vi "MeasLeakRate13.vi"() -> ()   [LabVIEW 2011]
panel:
  out "error out":errorcluster
  out "fit":cluster{"element":dbl, "Value":dbl}[](array[cluster])
  out "T-T0,P":cluster{"element":dbl, "element":dbl}[](array[cluster])
  out "t0":dbl format="%#_8f"
  out "XY Graph":T1(graph)
  out "S00":i32
  out "S20":dbl
  out "S11":dbl
  out "S10":dbl
  out "S01":dbl
  out "T,P":cluster{"element":dbl, "element":dbl}[](array[cluster])
  out "dPdt":dbl
  out "P0":dbl
  out "average P (Torr)":string
  in  "Control Valve local":bool
  in  "Exhaust Local":bool
  in  "Exhaust Close":bool
  in  "Exhaust Open":bool
  in  "Control Close":bool
  in  "Control Open":bool
  in  "reset":bool
  in  "# points to watch":i32=60
  out "leak rate (Torr/min)":string
  out "P":dbl
  out "first":bool=TRUE
  in  "interval (s)":dbl=0.5
  in  "stop":bool
  out "P(Torr)":string
  # "Pressure control valve:"
  # "Exahaust valve:"
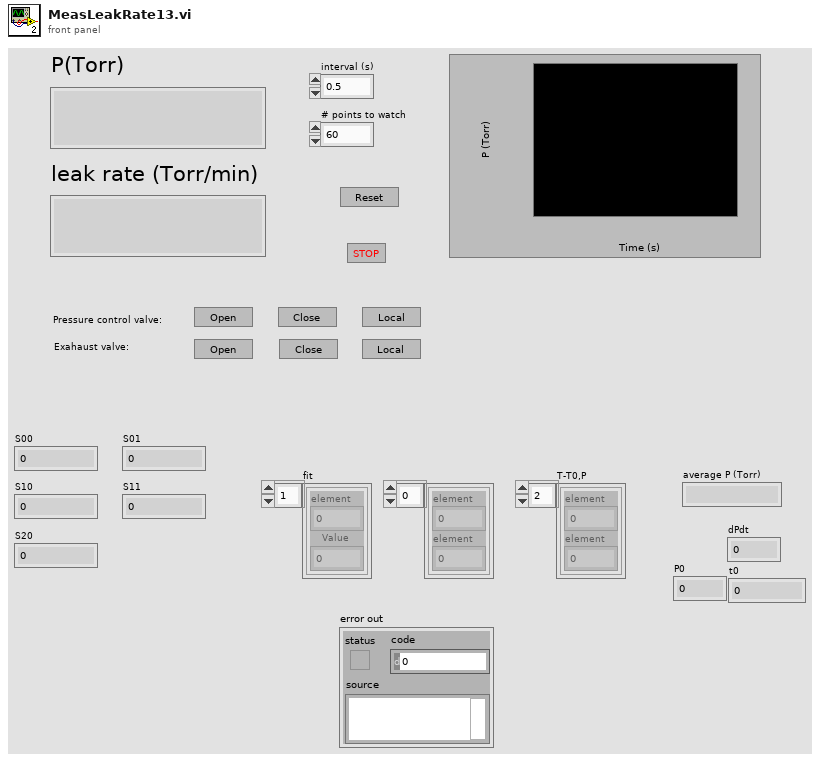
[diagram p1: front panel]
types:
  T1 = cluster{"Value":cluster{"element":dbl, "element":dbl}[]}[]
  T2 = cluster{"Value":cluster{"element":dbl, "Value":dbl}[]}[]
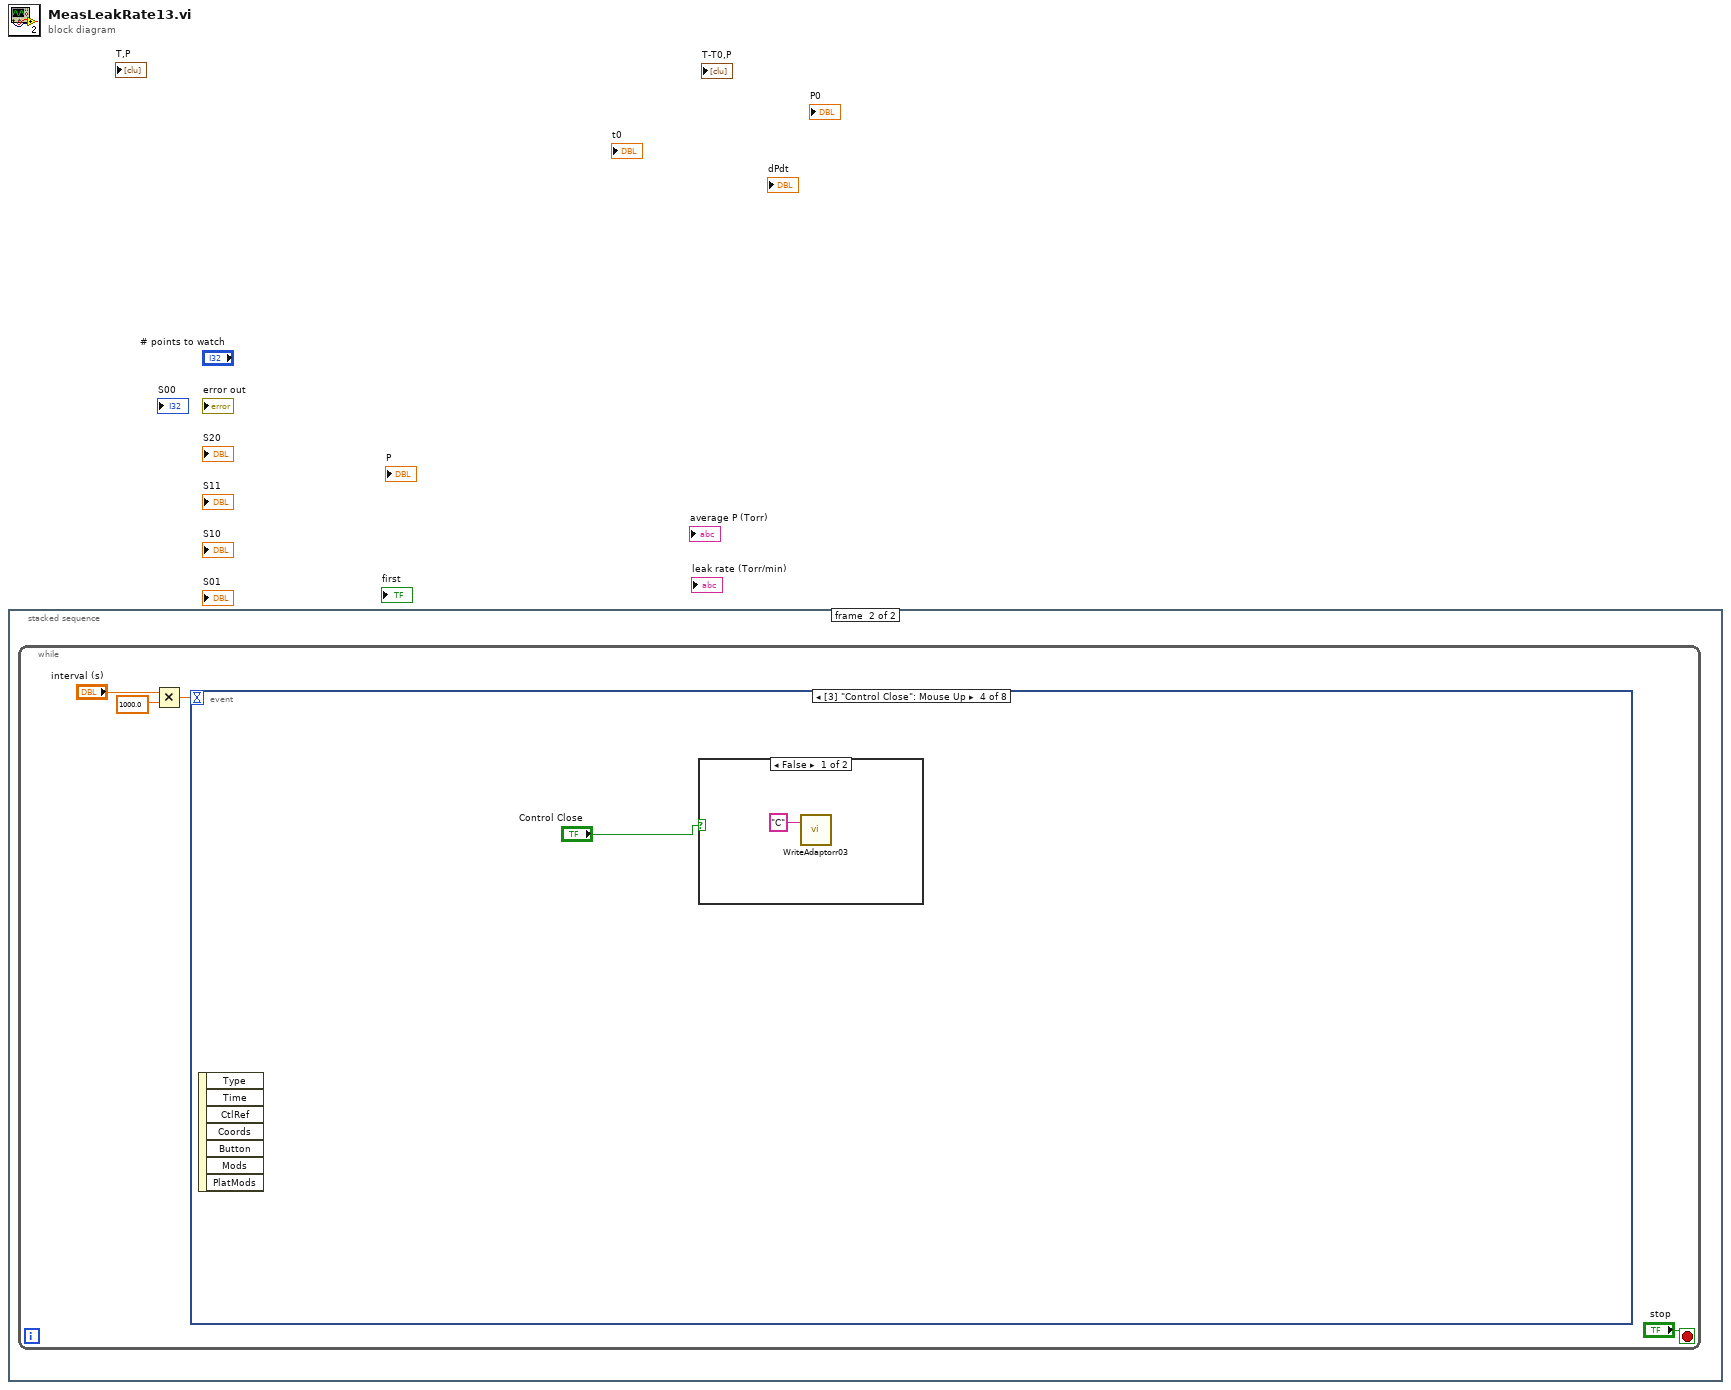
[diagram p0: block diagram]
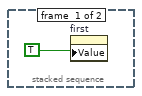
[diagram p2: hidden frame]
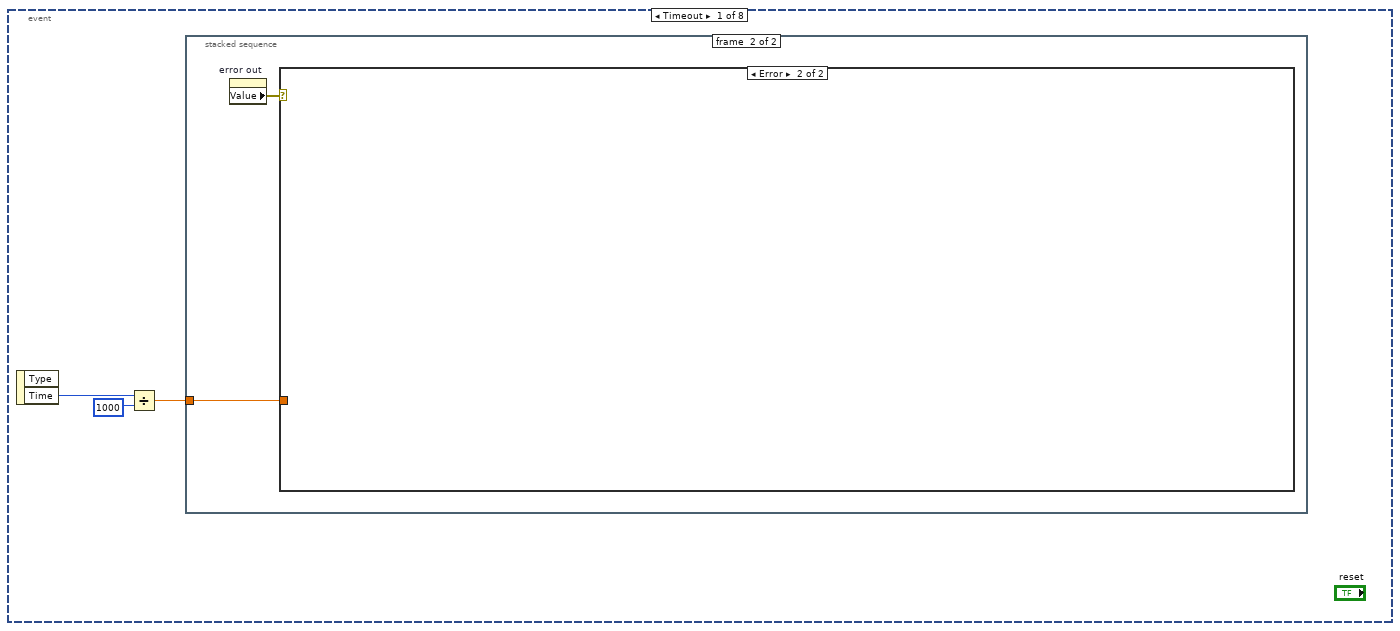
[diagram p3: hidden frame]
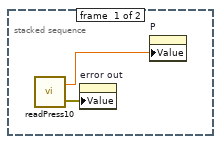
[diagram p4: hidden frame]
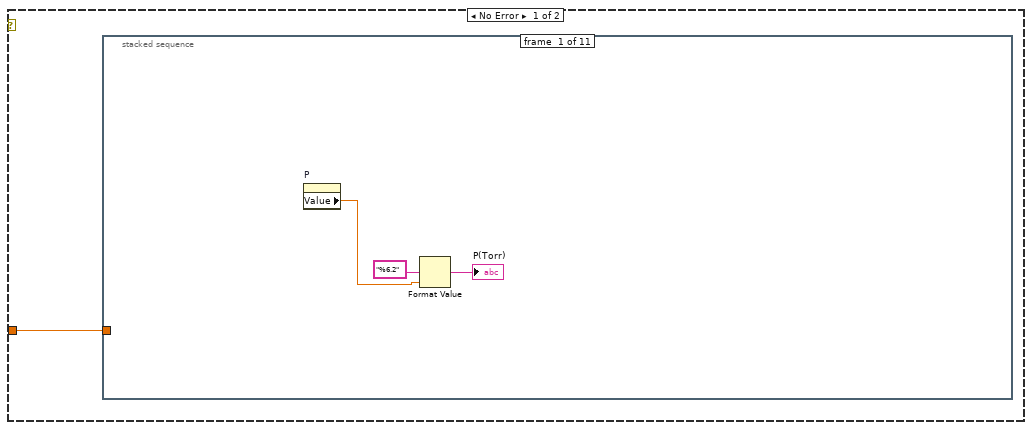
[diagram p5: hidden frame]
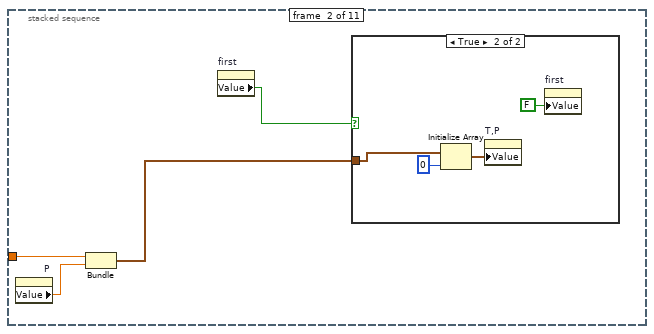
[diagram p6: hidden frame]
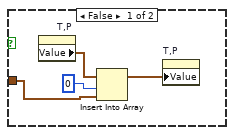
[diagram p7: hidden frame]
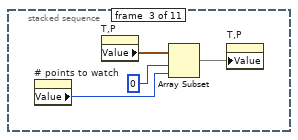
[diagram p8: hidden frame]
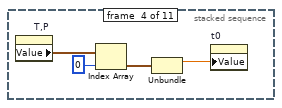
[diagram p9: hidden frame]
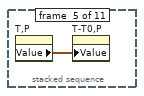
[diagram p10: hidden frame]
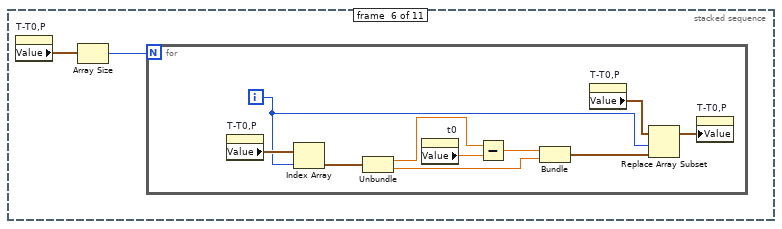
[diagram p11: hidden frame]
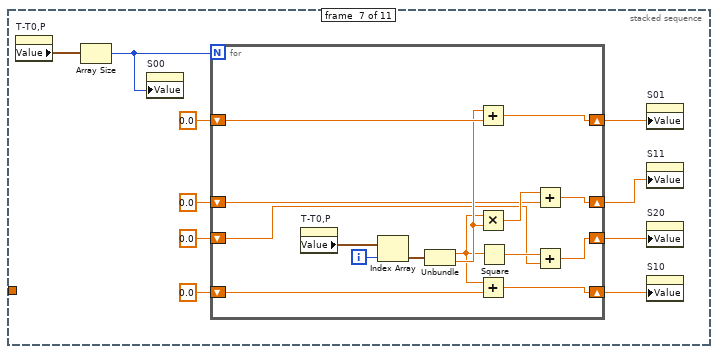
[diagram p12: hidden frame]
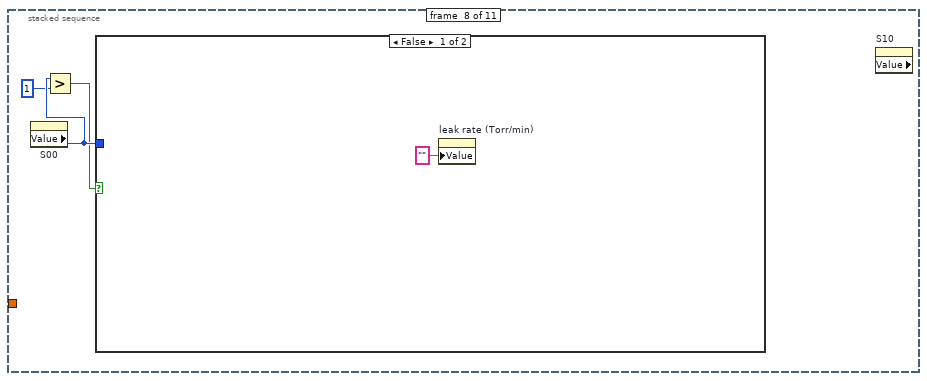
[diagram p13: hidden frame]
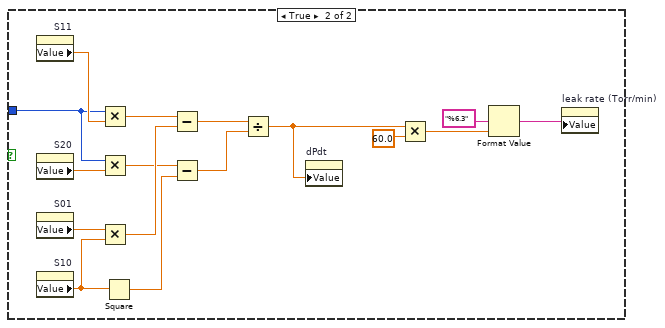
[diagram p14: hidden frame]
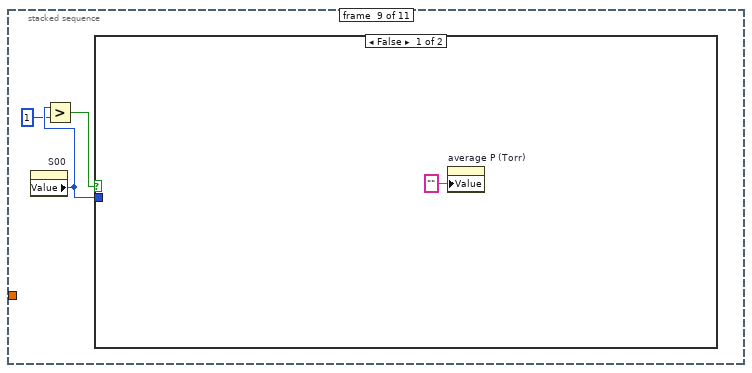
[diagram p15: hidden frame]
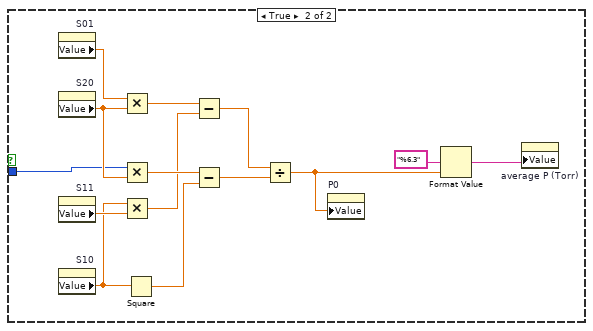
[diagram p16: hidden frame]
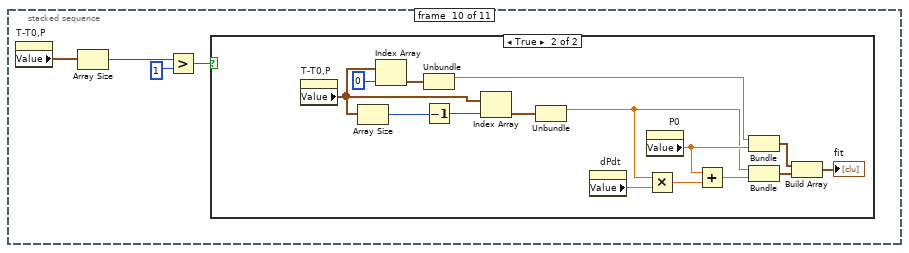
[diagram p17: hidden frame]
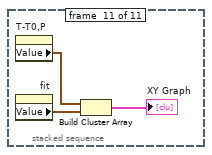
[diagram p19: hidden frame]
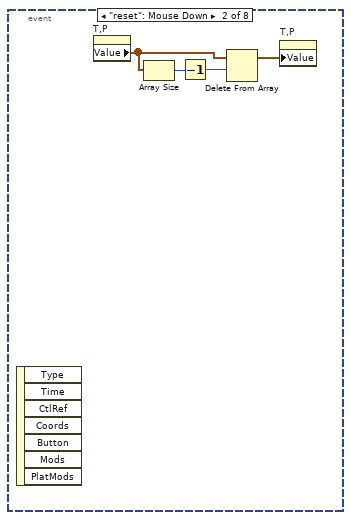
[diagram p20: hidden frame]
diagram:
  n1 = stacked-sequence {
    frame #0 {
      n2 = property on="first" class="Bool (strict)"("Value"=TRUE ("first")) -> ()  [unwired: 2 in, 2 out]
    }
    frame #1 {
      n3 = while {
        stop <- "stop" stop-if-true
        n4 = Multiply(x="interval (s)", y=1000.0) -> (x*y=w3:dbl)
        n5 = event shown="[3] \"Control Close\": Mouse Up" {
          selector: _ -> [_ _ _ _ _ _ _ _]
          dyn-events: _ -> [_ _ _ _ _ _ _ _]
          timeout: w3 -> [_ _ _ _ _ _ _ _]
          event Timeout {
            n6 = event-data() -> ("Time"=w8:u32)  [unwired: 1 in, 1 out]
            n7 = Divide(x=w8, y=u32 1000) -> (x/y=w6:dbl)
            n8 = stacked-sequence {
              tunnel: w6 -> [_ w11]
              frame #0 {
                n9 = call "readPress10.vi"() -> ("P"=w10:dbl, "error out"=w9:errorcluster)  [unwired: 1 in]
                n10 = property on="error out" class="Clust (strict)"("Value"=w9) -> ()  [unwired: 2 in, 2 out]
                n11 = property on="P" class="DigNum (strict)"("Value"=w10) -> ()  [unwired: 2 in, 2 out]
              }
              frame #1 {
                n12 = property on="error out" class="Clust (strict)"() -> ("Value"=w12:errorcluster)  [unwired: 2 in, 2 out]
                n13 = case shown="Error" w12 {
                  tunnel: w11 -> [w13 _]
                  frame No Error {
                    n14 = stacked-sequence {
                      tunnel: w13 -> [_ w19 _ _ _ _ _ _ _ _ _]
                      frame #0 {
                        n15 = property on="P" class="DigNum (strict)"() -> ("Value"=w14:dbl)  [unwired: 2 in, 2 out]
                        n16 = Format Value(format string="%6.2", value (0)=w14) -> (output string=→"P(Torr)":string)  [unwired: 1 in]
                      }
                      frame #1 {
                        n17 = property on="P" class="DigNum (strict)"() -> ("Value"=w20:dbl)  [unwired: 2 in, 2 out]
                        n18 = Bundle(w19, "Value"=w20) -> (w18:cluster{dbl, "Value":dbl})  [unwired: 1 in]
                        n19 = property on="first" class="Bool (strict)"() -> ("Value"=w17:bool)  [unwired: 2 in, 2 out]
                        n20 = case shown="True" w17 {
                          tunnel: w18 -> [w21 w26]
                          frame False {
                            n21 = property on="T,P" class="Arr (strict)"() -> ("Value"=w22:cluster{"element":dbl, "element":dbl}[])  [unwired: 2 in, 2 out]
                            n22 = Insert Into Array(array=w22, index=0, new element=w21) -> (w24:cluster{"element":dbl, "element":dbl}[])
                            n23 = property on="T,P" class="Arr (strict)"("Value"=w24) -> ()  [unwired: 2 in, 2 out]
                          }
                          frame True {
                            n24 = Initialize Array(w26, 0 ("dimension size")) -> (w27:cluster{dbl, "Value":dbl}[])
                            n25 = property on="T,P" class="Arr (strict)"("Value"=w27) -> ()  [unwired: 2 in, 2 out]
                            n26 = property on="first" class="Bool (strict)"("Value"=FALSE ("first")) -> ()  [unwired: 2 in, 2 out]
                          }
                        }
                      }
                      frame #2 {
                        n27 = property on="# points to watch" class="DigNum (strict)"() -> ("Value"=w30:i32)  [unwired: 2 in, 2 out]
                        n28 = property on="T,P" class="Arr (strict)"() -> ("Value"=w31:cluster{"element":dbl, "element":dbl}[])  [unwired: 2 in, 2 out]
                        n29 = Array Subset(array=w31, index=0, length=w30) -> (w29:cluster{"element":dbl, "element":dbl}[])
                        n30 = property on="T,P" class="Arr (strict)"("Value"=w29) -> ()  [unwired: 2 in, 2 out]
                      }
                      frame #3 {
                        n31 = property on="T,P" class="Arr (strict)"() -> ("Value"=w36:cluster{"element":dbl, "element":dbl}[])  [unwired: 2 in, 2 out]
                        n32 = Index Array(array=w36, index=0) -> (element=w34:cluster{"element":dbl, "element":dbl})
                        n33 = Unbundle(w34) -> ("element"=w33:dbl)  [unwired: 1 out]
                        n34 = property on="t0" class="DigNum (strict)"("Value"=w33) -> ()  [unwired: 2 in, 2 out]
                      }
                      frame #4 {
                        n35 = property on="T,P" class="Arr (strict)"() -> ("Value"=w37:cluster{"element":dbl, "element":dbl}[])  [unwired: 2 in, 2 out]
                        n36 = property on="T-T0,P" class="Arr (strict)"("Value"=w37) -> ()  [unwired: 2 in, 2 out]
                      }
                      frame #5 {
                        n37 = property on="T-T0,P" class="Arr (strict)"() -> ("Value"=w39:cluster{"element":dbl, "element":dbl}[])  [unwired: 2 in, 2 out]
                        n38 = Array Size(array=w39) -> (size(s)=w38:i32)
                        n39 = for {
                          N: w38 -> [_]
                          i -> [w40]
                          n40 = property on="T-T0,P" class="Arr (strict)"() -> ("Value"=w44:cluster{"element":dbl, "element":dbl}[])  [unwired: 2 in, 2 out]
                          n41 = Index Array(array=w44, index=w40) -> (element=w49:cluster{"element":dbl, "element":dbl})
                          n42 = Unbundle(w49) -> ("element"=w48:dbl, "element"=w45:dbl)
                          n43 = property on="t0" class="DigNum (strict)"() -> ("Value"=w47:dbl)  [unwired: 2 in, 2 out]
                          n44 = Subtract(x=w48, y=w47) -> (x-y=w46:dbl)
                          n45 = Bundle(w46, "element"=w45) -> (w43:cluster{dbl, "element":dbl})  [unwired: 1 in]
                          n46 = property on="T-T0,P" class="Arr (strict)"() -> ("Value"=w42:cluster{"element":dbl, "element":dbl}[])  [unwired: 2 in, 2 out]
                          n47 = Replace Array Subset(array=w42, new element=w43, index=w40) -> (w41:cluster{"element":dbl, "element":dbl}[])
                          n48 = property on="T-T0,P" class="Arr (strict)"("Value"=w41) -> ()  [unwired: 2 in, 2 out]
                        }
                      }
                      frame #6 {
                        n49 = property on="T-T0,P" class="Arr (strict)"() -> ("Value"=w50:cluster{"element":dbl, "element":dbl}[])  [unwired: 2 in, 2 out]
                        n50 = Array Size(array=w50) -> (size(s)=w54:i32)
                        n51 = property on="S00" class="DigNum (strict)"("Value"=w54) -> ()  [unwired: 2 in, 2 out]
                        n52 = for {
                          N: w54 -> [_]
                          shift-right: [w72] -> w53
                          shift-left: 0.0 -> [w74]
                          shift-right: [w71] -> w57
                          shift-left: 0.0 -> [w70]
                          shift-right: [w67] -> w52
                          shift-left: 0.0 -> [w66]
                          shift-right: [w63] -> w51
                          shift-left: 0.0 -> [w62]
                          i -> [w61]
                          n53 = property on="T-T0,P" class="Arr (strict)"() -> ("Value"=w60:cluster{"element":dbl, "element":dbl}[])  [unwired: 2 in, 2 out]
                          n54 = Index Array(array=w60, index=w61) -> (element=w73:cluster{"element":dbl, "element":dbl})
                          n55 = Unbundle(w73) -> ("element"=w65:dbl, "element"=w69:dbl)
                          n56 = Add(x=w69, y=w70) -> (x+y=w71:dbl)
                          n57 = Multiply(x=w65, y=w69) -> (x*y=w68:dbl)
                          n58 = Add(x=w65, y=w74) -> (x+y=w72:dbl)
                          n59 = Square(x=w65) -> (x^2=w64:dbl)
                          n60 = Add(x=w68, y=w66) -> (x+y=w67:dbl)
                          n61 = Add(x=w64, y=w62) -> (x+y=w63:dbl)
                        }
                        n62 = property on="S01" class="DigNum (strict)"("Value"=w57) -> ()  [unwired: 2 in, 2 out]
                        n63 = property on="S11" class="DigNum (strict)"("Value"=w52) -> ()  [unwired: 2 in, 2 out]
                        n64 = property on="S20" class="DigNum (strict)"("Value"=w51) -> ()  [unwired: 2 in, 2 out]
                        n65 = property on="S10" class="DigNum (strict)"("Value"=w53) -> ()  [unwired: 2 in, 2 out]
                      }
                      frame #7 {
                        n66 = property on="S00" class="DigNum (strict)"() -> ("Value"=w77:i32)  [unwired: 2 in, 2 out]
                        n67 = Greater?(x=w77, y=1) -> (0:w75:bool)
                        n68 = case shown="False" w75 {
                          tunnel: w77 -> [_ w82]
                          frame False {
                            n69 = property on="leak rate (Torr/min)" class="Str"("Value"="" ("leak rate (Torr/min)")) -> ()  [unwired: 2 in, 2 out]
                          }
                          frame True {
                            n70 = property on="S11" class="DigNum (strict)"() -> ("Value"=w84:dbl)  [unwired: 2 in, 2 out]
                            n71 = property on="S20" class="DigNum (strict)"() -> ("Value"=w83:dbl)  [unwired: 2 in, 2 out]
                            n72 = property on="S01" class="DigNum (strict)"() -> ("Value"=w81:dbl)  [unwired: 2 in, 2 out]
                            n73 = property on="S10" class="DigNum (strict)"() -> ("Value"=w85:dbl)  [unwired: 2 in, 2 out]
                            n74 = Multiply(x=w82, y=w84) -> (x*y=w94:dbl)
                            n75 = Multiply(x=w82, y=w83) -> (x*y=w92:dbl)
                            n76 = Multiply(x=w81, y=w85) -> (x*y=w93:dbl)
                            n77 = Square(x=w85) -> (x^2=w91:dbl)
                            n78 = Subtract(x=w94, y=w93) -> (x-y=w90:dbl)
                            n79 = Subtract(x=w92, y=w91) -> (x-y=w89:dbl)
                            n80 = Divide(x=w90, y=w89) -> (x/y=w80:dbl)
                            n81 = property on="dPdt" class="DigNum (strict)"("Value"=w80) -> ()  [unwired: 2 in, 2 out]
                            n82 = Multiply(x=w80, y=60.0) -> (x*y=w86:dbl)
                            n83 = Format Value(format string="%6.3", value (0)=w86) -> (output string=w79:string)  [unwired: 1 in]
                            n84 = property on="leak rate (Torr/min)" class="Str"("Value"=w79) -> ()  [unwired: 2 in, 2 out]
                          }
                        }
                        n85 = property on="S10" class="DigNum (strict)" props=["Value"]() -> ()  [unwired: 2 in, 3 out]
                      }
                      frame #8 {
                        n86 = property on="S00" class="DigNum (strict)"() -> ("Value"=w97:i32)  [unwired: 2 in, 2 out]
                        n87 = Greater?(x=w97, y=1) -> (0:w95:bool)
                        n88 = case shown="False" w95 {
                          tunnel: w97 -> [_ w100]
                          frame False {
                            n89 = property on="average P (Torr)" class="Str"("Value"="" ("average P (Torr)")) -> ()  [unwired: 2 in, 2 out]
                          }
                          frame True {
                            n90 = property on="S01" class="DigNum (strict)"() -> ("Value"=w112:dbl)  [unwired: 2 in, 2 out]
                            n91 = property on="S20" class="DigNum (strict)"() -> ("Value"=w109:dbl)  [unwired: 2 in, 2 out]
                            n92 = property on="S11" class="DigNum (strict)"() -> ("Value"=w111:dbl)  [unwired: 2 in, 2 out]
                            n93 = property on="S10" class="DigNum (strict)"() -> ("Value"=w110:dbl)  [unwired: 2 in, 2 out]
                            n94 = Multiply(x=w112, y=w109) -> (x*y=w102:dbl)
                            n95 = Multiply(x=w100, y=w109) -> (x*y=w105:dbl)
                            n96 = Multiply(x=w110, y=w111) -> (x*y=w101:dbl)
                            n97 = Square(x=w110) -> (x^2=w104:dbl)
                            n98 = Subtract(x=w102, y=w101) -> (x-y=w108:dbl)
                            n99 = Subtract(x=w105, y=w104) -> (x-y=w103:dbl)
                            n100 = Divide(x=w108, y=w103) -> (x/y=w106:dbl)
                            n101 = property on="P0" class="DigNum (strict)"("Value"=w106) -> ()  [unwired: 2 in, 2 out]
                            n102 = Format Value(format string="%6.3", value (0)=w106) -> (output string=w99:string)  [unwired: 1 in]
                            n103 = property on="average P (Torr)" class="Str"("Value"=w99) -> ()  [unwired: 2 in, 2 out]
                          }
                        }
                      }
                      frame #9 {
                        n104 = property on="T-T0,P" class="Arr (strict)"() -> ("Value"=w116:cluster{"element":dbl, "element":dbl}[])  [unwired: 2 in, 2 out]
                        n105 = Array Size(array=w116) -> (size(s)=w115:i32)
                        n106 = Greater?(x=w115, y=1) -> (0:w113:bool)
                        n107 = case shown="True" w113 {
                          frame False {
                          }
                          frame True {
                            n108 = property on="T-T0,P" class="Arr (strict)"() -> ("Value"=w120:cluster{"element":dbl, "element":dbl}[])  [unwired: 2 in, 2 out]
                            n109 = Array Size(array=w120) -> (size(s)=w130:i32)
                            n110 = Index Array(array=w120, index=0) -> (element=w128:cluster{"element":dbl, "element":dbl})
                            n111 = Unbundle(w128) -> ("element"=w123:dbl)  [unwired: 1 out]
                            n112 = Decrement(x=w130) -> (x-1=w129:i32)
                            n113 = Index Array(array=w120, index=w129) -> (element=w127:cluster{"element":dbl, "element":dbl})
                            n114 = Unbundle(w127) -> ("element"=w121:dbl)  [unwired: 1 out]
                            n115 = property on="dPdt" class="DigNum (strict)"() -> ("Value"=w126:dbl)  [unwired: 2 in, 2 out]
                            n116 = property on="P0" class="DigNum (strict)"() -> ("Value"=w124:dbl)  [unwired: 2 in, 2 out]
                            n117 = Multiply(x=w121, y=w126) -> (x*y=w125:dbl)
                            n118 = Add(x=w124, y=w125) -> (x+y=w122:dbl)
                            n119 = Bundle("element"=w123, "Value"=w124) -> (w119:cluster{"element":dbl, "Value":dbl})  [unwired: 1 in]
                            n120 = Bundle("element"=w121, w122) -> (w118:cluster{"element":dbl, dbl})  [unwired: 1 in]
                            n121 = Build Array(w119, w118) -> (→"fit":cluster{"element":dbl, "Value":dbl}[])
                          }
                        }
                      }
                      frame #10 {
                        n122 = property on="T-T0,P" class="Arr (strict)"() -> ("Value"=w134:cluster{"element":dbl, "element":dbl}[])  [unwired: 2 in, 2 out]
                        n123 = property on="fit" class="Arr (strict)"() -> ("Value"=w132:cluster{"element":dbl, "Value":dbl}[])  [unwired: 2 in, 2 out]
                        n124 = Build Cluster Array(w134, w132) -> (→"XY Graph":T2)
                      }
                    }
                  }
                  frame Error {
                  }
                }
              }
            }
          }
          event "reset": Mouse Down {
            n125 = event-data() -> ()  [unwired: 1 in, 7 out]
            n126 = property on="T,P" class="Arr (strict)"() -> ("Value"=w136:cluster{"element":dbl, "element":dbl}[])  [unwired: 2 in, 2 out]
            n127 = Array Size(array=w136) -> (size(s)=w138:i32)
            n128 = Decrement(x=w138) -> (x-1=w137:i32)
            n129 = Delete From Array(array=w136, length=w137) -> (array with subset deleted=w135:cluster{"element":dbl, "element":dbl}[])  [unwired: 1 in, 1 out]
            n130 = property on="T,P" class="Arr (strict)"("Value"=w135) -> ()  [unwired: 2 in, 2 out]
          }
          event "Control Open": Mouse Up {
            n131 = event-data() -> ()  [unwired: 1 in, 7 out]
            n132 = case shown="False" "Control Open" {
              frame False {
                n133 = call "WriteAdaptorr03.vi"("string to write"="O") -> ()  [unwired: 1 in, 1 out]
              }
              frame True {
              }
            }
          }
          event "Control Close": Mouse Up {
            n134 = event-data() -> ()  [unwired: 1 in, 7 out]
            n135 = case shown="False" "Control Close" {
              frame False {
                n136 = call "WriteAdaptorr03.vi"("string to write"="C") -> ()  [unwired: 1 in, 1 out]
              }
              frame True {
              }
            }
          }
          event "Exhaust Open": Mouse Up {
            n137 = event-data() -> ()  [unwired: 1 in, 7 out]
            n138 = case shown="True" "Exhaust Open" {
              frame False {
              }
              frame True {
                n139 = call "set_vacuum.vi"("Vac Remote"=TRUE, "Atm Exhaust"=FALSE, "Vac Exhaust"=TRUE) -> ()
              }
            }
          }
          event "Exhaust Close": Mouse Up {
            n140 = event-data() -> ()  [unwired: 1 in, 7 out]
            n141 = case shown="True" "Exhaust Close" {
              frame False {
              }
              frame True {
                n142 = call "set_vacuum.vi"("Vac Remote"=TRUE, "Atm Exhaust"=FALSE, "Vac Exhaust"=FALSE) -> ()
              }
            }
          }
          event "Exhaust Local": Mouse Up {
            n143 = event-data() -> ()  [unwired: 1 in, 7 out]
            n144 = case shown="True" "Exhaust Local" {
              frame False {
              }
              frame True {
                n145 = call "set_vacuum.vi"() -> ()  [unwired: 3 in]
              }
            }
          }
          event "Control Valve local": Mouse Down? {
            n146 = event-data() -> ()  [unwired: 1 in, 7 out]
            n147 = case shown="False" "Control Valve local" {
              frame False {
                n148 = call "WriteAdaptorr03.vi"("string to write"="D5") -> ()  [unwired: 1 in, 1 out]
              }
              frame True {
              }
            }
            n149 = event-data() -> ()  [unwired: 5 in, 1 out]
          }
        }
      }
    }
  }
